vi "Comments.Add Lockin Description.vi"(7 "error in (no error)":errorcluster, 10 "Control Experiment":refnum<class "Control Experiment.lvclass">) -> (0 "error out":errorcluster, 3 "Control Experiment out":refnum<class "Control Experiment.lvclass">)   [LabVIEW 2016, in "Control Experiment.lvclass"]
uses:
  Control Experiment.lvclass
  Control Experiment.lvclass/Control Experiment.ctl
  <userlib>/LevyLab/PLYM/YAML.lvclass
panel:
  out "Lockin Comments":string
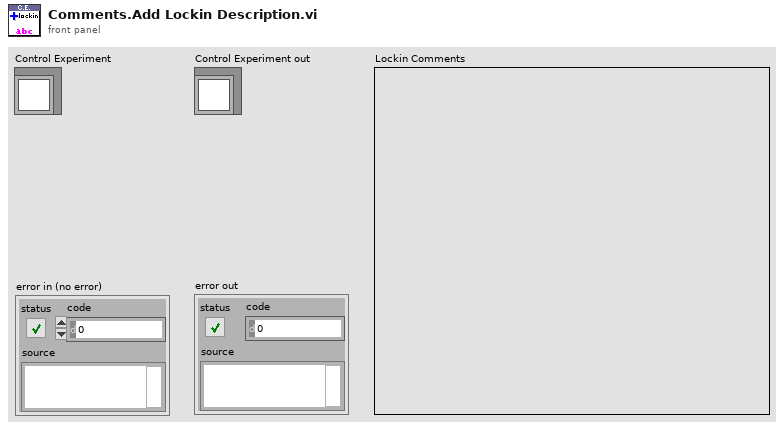
[diagram p1: front panel]
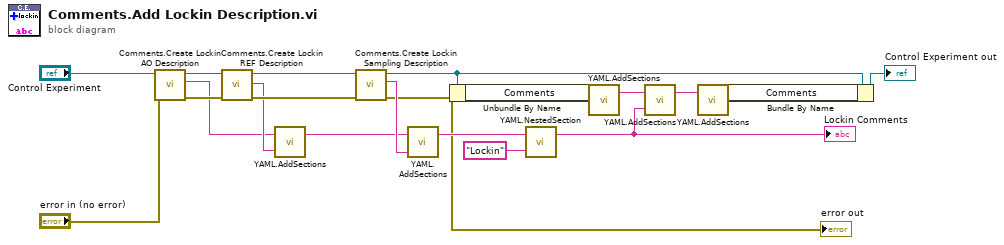
[diagram p0: block diagram]
diagram:
  n1 = call "Comments.Create Lockin AO Description.vi"("error in (no error)"="error in (no error)", "Control Experiment"="Control Experiment") -> ("error out"=w14:errorcluster, "AO Section"=w6:string, "Control Experiment out"=w15:refnum<class "Control Experiment.lvclass">)  [unwired: 6 in]
  n2 = call "Comments.Create Lockin REF Description.vi"("error in (no error)"=w14, "Control Experiment"=w15) -> ("error out"=w12:errorcluster, "REF Section"=w8:string, "Control Experiment out"=w13:refnum<class "Control Experiment.lvclass">)  [unwired: 6 in]
  n3 = call <userlib>:"YAML.AddSections.vi"("Section 2"=w8, "Section 1"=w6) -> ("Output"=w7:string)  [unwired: 1 in]
  n4 = call "Comments.Create Lockin Sampling Description.vi"("error in (no error)"=w12, "Control Experiment"=w13) -> ("error out"=→"error out":errorcluster, "Sampling Section"=w9:string, "Control Experiment out"=w16:refnum<class "Control Experiment.lvclass">)  [unwired: 6 in]
  n5 = call <userlib>:"YAML.AddSections.vi"("Section 2"=w9, "Section 1"=w7) -> ("Output"=w5:string)  [unwired: 1 in]
  n6 = Unbundle By Name(w16) -> ("Comments"=w19:string)
  n7 = call <userlib>:"YAML.NestedSection.vi"("Section Key"="Lockin" ("string"), "Nested Section"=w5) -> ("String"=w10:string)  [unwired: 1 in]
  "Lockin Comments" <- w10
  n8 = call <userlib>:"YAML.AddSections.vi"("Section 1"=w19) -> ("Output"=w18:string)  [unwired: 2 in]
  n9 = call <userlib>:"YAML.AddSections.vi"("Section 2"=w10, "Section 1"=w18) -> ("Output"=w2:string)  [unwired: 1 in]
  n10 = call <userlib>:"YAML.AddSections.vi"("Section 1"=w2) -> ("Output"=w1:string)  [unwired: 2 in]
  n11 = Bundle By Name(cluster=w16, "Comments"=w1) -> (→"Control Experiment out":refnum<class "Control Experiment.lvclass">)
